vi "FindParticlesWrapper.vi"(7 "?":T1, 8 "error in":errorcluster, 9 "Settings":T5={"Harware Configuration"={"Camera"="cam1", "Frames Per Second"=15, "Simulate Recording"=FALSE, "Simulated Recording Sample"=path "", "Timestamp Method"=enum."Camera Timestamp"}, "Base Recording Path"=path "", "Type Of Recording"="", "Recording Codec"="", "TrackingSettings"={"Max Radius"=0, "Threshold"=255.0, "ROI"={"Left"=1, "Top"=1, "Right"=2, "Bottom"=0, "Rotation"=0.0}}, "Calibration"={"Pixel Width (X)"=1.0, "Pixel Height (Y)"=1.0}, "Broadcast Length"=0} {"Broadcast Length" min=0; "TrackingSettings"."ROI"."Rotation" format="%.2f"; "TrackingSettings"."ROI"."Left" scale=0.0..1024.0; "TrackingSettings"."ROI"."Right" scale=0.0..1024.0; "TrackingSettings"."Threshold" scale=0.0..255.0}, 10 "Data Old":T3 {"Frame Data"."Image Type" items=["Grayscale (U8)", "Grayscale (I16)", "Grayscale (SGL)", "Complex (CSG)", "RGB (U32)", "HSL (U32)", "RGB (U64)", "Grayscale (U16)"]}, 11 "Data":T3 {"Frame Data"."Image Type" items=["Grayscale (U8)", "Grayscale (I16)", "Grayscale (SGL)", "Complex (CSG)", "RGB (U32)", "HSL (U32)", "RGB (U64)", "Grayscale (U16)"]}) -> (0 "error out":errorcluster, 3 "Data Out":T3 {"Frame Data"."Image Type" items=["Grayscale (U8)", "Grayscale (I16)", "Grayscale (SGL)", "Complex (CSG)", "RGB (U32)", "HSL (U32)", "RGB (U64)", "Grayscale (U16)"]}, 5 "?":T1)   [LabVIEW 2017, in "ImageAcquisitionLibrary.lvlib"]
uses:
  ImageAcquisitionLibrary.lvlib
  Settings/Settings.ctl
  <vilib>/userdefined/High Color/IMAQdx.ctl
  TrackingSettings.ctl
  Settings/Calibration.ctl
  Acquisition/AcquireData.ctl
  TrackingImages.ctl
  <vilib>/vision/Image Controls.llb/IMAQ Image.ctl
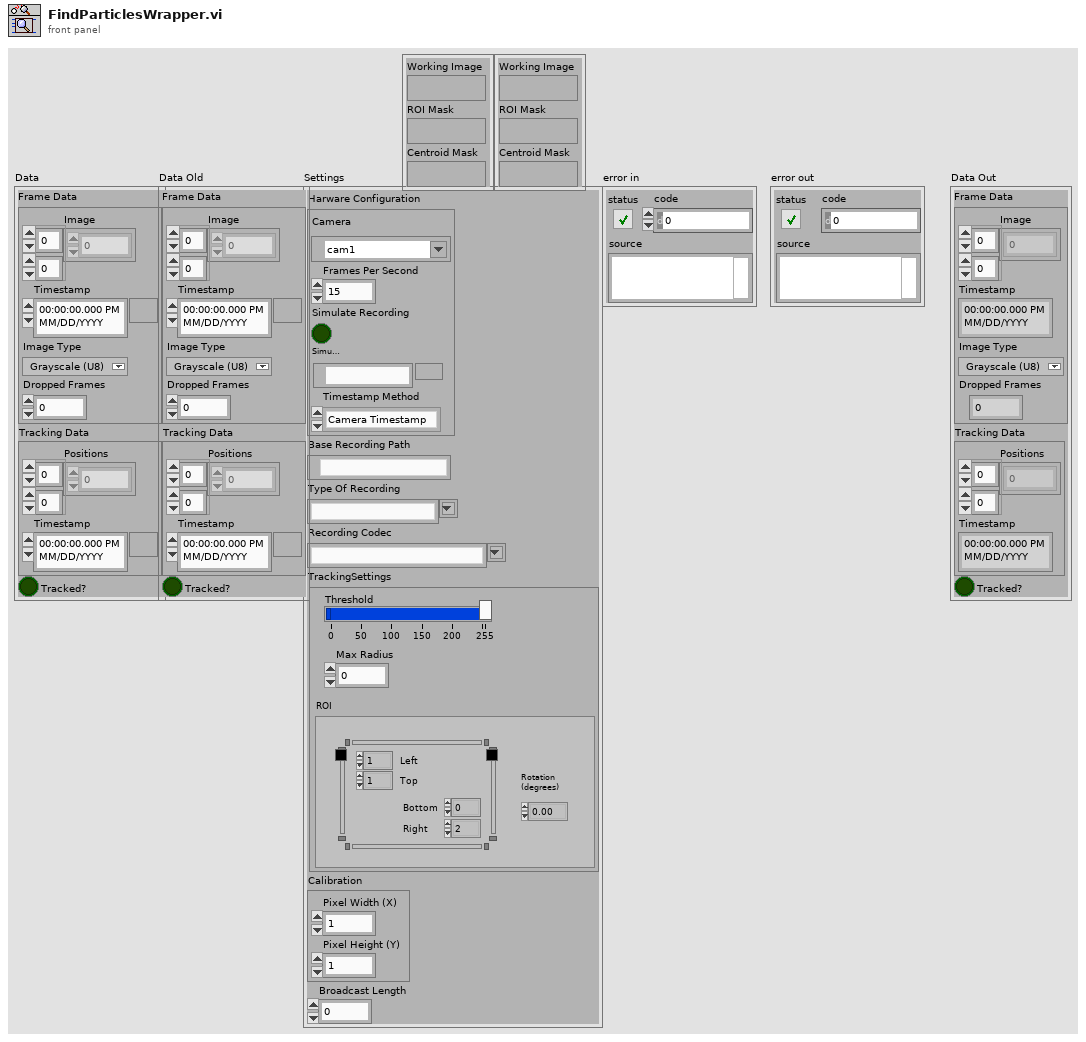
[diagram p1: front panel]
types:
  T1 = typedef "ImageAcquisitionLibrary.lvlib/TrackingImages.ctl" = cluster{"Working Image":T2, "ROI Mask":T2, "Centroid Mask":T2}
  T2 = typedef "IMAQ Image.ctl" = refnum<image>
  T3 = typedef "ImageAcquisitionLibrary.lvlib/AcquireData.ctl" = cluster{"Frame Data":cluster{"Image":u32[][], "Timestamp":timestamp, "Image Type":T4, "Dropped Frames":u32}, "Tracking Data":cluster{"Positions":dbl[][], "Timestamp":timestamp}, "Tracked?":bool}
  T4 = typedef "Image Type" = u32
  T5 = typedef "ImageAcquisitionLibrary.lvlib/Settings.ctl" = cluster{"Harware Configuration":cluster{"Camera":T6, "Frames Per Second":u32, "Simulate Recording":bool, "Simulated Recording Sample":path, "Timestamp Method":enum16{"System Timestamp", "Camera Timestamp", "IMAQdx Timestamp"}}, "Base Recording Path":path, "Type Of Recording":string, "Recording Codec":string, "TrackingSettings":T7, "Calibration":T9, "Broadcast Length":i32}
  T6 = typedef "IMAQdx.ctl" = refnum<k21>
  T7 = typedef "ImageAcquisitionLibrary.lvlib/TrackingSettings.ctl" = cluster{"Max Radius":i32, "Threshold":sgl, "ROI":T8}
  T8 = typedef "IMAQ Rectangle" = cluster{"Left":i32, "Top":i32, "Right":i32, "Bottom":i32, "Rotation":dbl}
  T9 = typedef "ImageAcquisitionLibrary.lvlib/Calibration.ctl" = cluster{"Pixel Width (X)":dbl, "Pixel Height (Y)":dbl}
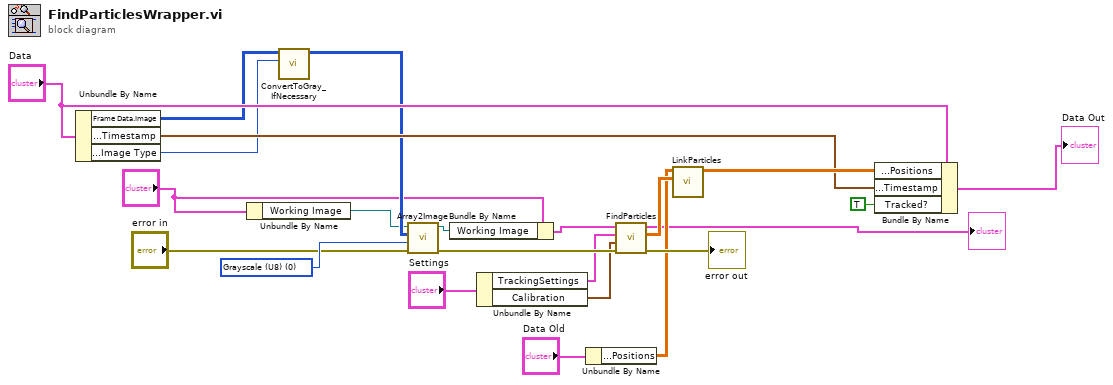
[diagram p0: block diagram]
diagram:
  w13 = T4 0 items=["Grayscale (U8)", "Grayscale (I16)", "Grayscale (SGL)", "Complex (CSG)", "RGB (U32)", "HSL (U32)", "RGB (U64)", "Grayscale (U16)"] ("Image Type")
  n1 = Unbundle By Name("Data") -> ("Frame Data.Image"=w12:u32[][], "Frame Data.Timestamp"=w15:timestamp, "Frame Data.Image Type"=w3:T4)
  n2 = Unbundle By Name("?") -> ("Working Image"=w8:T2)
  n3 = call "ConvertToGray_IfNecessary.vi"("Image Type"=w3, "Image in"=w12) -> ("Image out"=w11:u32[][])  [unwired: 9 in]
  n4 = call "Array2Image.vi"("error in (no error)"="error in", "Image Type"=w13, "Image Pixels (U32)"=w11, "Image 2"=w8) -> ("error out"=w10:errorcluster, "Image"=w6:T2)  [unwired: 6 in]
  n5 = Bundle By Name(cluster="?", "Working Image"=w6) -> (w1:T1)
  n6 = Unbundle By Name("Settings") -> ("TrackingSettings"=w7:T7, "Calibration"=w5:T9)
  n7 = Unbundle By Name("Data Old") -> ("Tracking Data.Positions"=w16:dbl[][])
  n8 = call "FindParticles.vi"("error in (no error)"=w10, "Calibration 2"=w5, "TrackingSettings"=w7, 11:w1) -> ("error out 2"=→"error out":errorcluster, "Centroids 2"=w19:dbl[][], 3:→"?":T1)  [unwired: 5 in]
  n9 = call "LinkParticles.vi"("New Particle Positions"=w19, "Old Particle Positions"=w16) -> ("New Particle Positions Out"=w18:dbl[][])  [unwired: 9 in]
  n10 = Bundle By Name(cluster="Data", "Tracking Data.Positions"=w18, "Tracking Data.Timestamp"=w15, "Tracked?"=TRUE) -> (→"Data Out":T3)
